vi "toggle.vi"(11 "In":bool) -> (3 "Out":bool)   [LabVIEW 2013]
panel:
  in  "Initial":bool
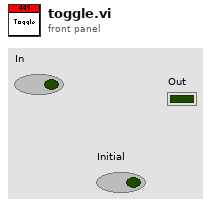
[diagram p1: front panel]
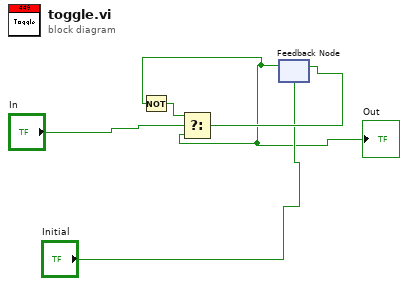
[diagram p0: block diagram]
diagram:
  n1 = feedback #1("Initial") -> (w1:bool)
  "Out" <- w1
  n2 = Not(x=w1) -> (.not. x?=w5:bool)
  n3 = Select(t=w5, s="In", f=w1) -> (s? t:f=w4:bool)
  n4 = feedback-in #1(w4) -> ()
